vi "Close.vi"(0 "Modbus master in":refnum<class "Modbus Master.lvclass">, 11 "error in (no error)":errorcluster) -> (15 "error out":errorcluster)   [LabVIEW 2024]
doc: "Close connection to slave Adams module."
uses:
  <vilib>/NI/Modbus Library/API/Master/Modbus Master.lvclass
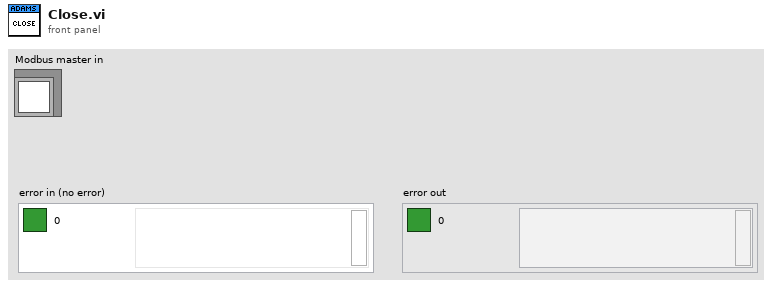
[diagram p1: front panel]
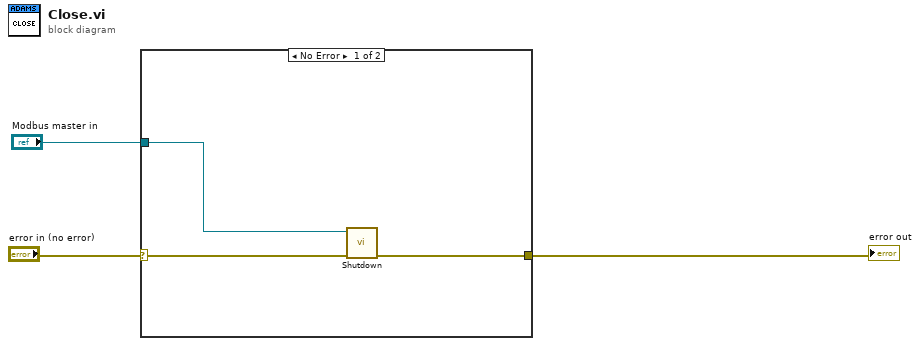
[diagram p0: block diagram]
diagram:
  n1 = case shown="No Error" "error in (no error)" {
    selector: "error in (no error)" -> [w6 w7]
    tunnel: "Modbus master in" -> [w5 _]
    tunnel: [w4 w7] -> w1
    frame No Error {
      n2 = call-dynamic "Shutdown.vi"("error in"=w6, "Modbus master in"=w5) -> ("error out"=w4:errorcluster)  [unwired: 9 in]
    }
    frame Error {
    }
  }
  "error out" <- w1
